vi "SIM_FrameProperties.vi"() -> (0 "data":dbl[][](array[numeric]), 3 "Frame Properties":T1)   [LabVIEW 2019]
uses:
  <vilib>/Utility/file.llb/Read Delimited Spreadsheet (DBL).vi
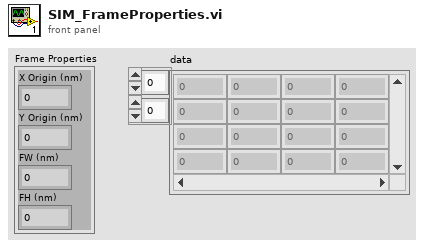
[diagram p1: front panel]
types:
  T1 = cluster{"X Origin (nm)":dbl, "Y Origin (nm)":dbl, "FW (nm)":dbl, "FH (nm)":dbl}
  T2 = cluster{"[0]":dbl, "[1]":dbl, "[2]":dbl, "[3]":dbl, "[4]":dbl, "[5]":dbl, "[6]":dbl, "[7]":dbl, "[8]":dbl}
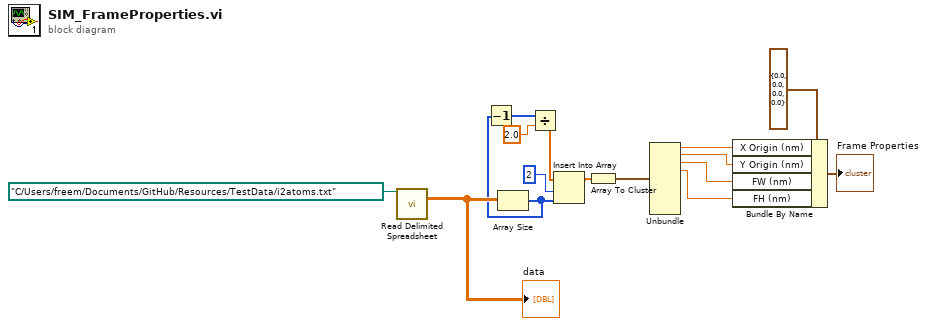
[diagram p0: block diagram]
diagram:
  n1 = call-poly <vilib>:"Read Delimited Spreadsheet.vi"("file path (dialog if empty)"=path "C:/Users/freem/Documents/GitHub/Resources/TestData/i2atoms.txt") -> ("all rows"=w14:dbl[][])  [unwired: 9 in, 5 out]
  "data" <- w14
  n2 = Array Size(array=w14) -> (size(s)=w2:i32[])
  n3 = Decrement(x=w2) -> (x-1=w4:i32[])
  n4 = Divide(x=w4, y=2.0) -> (x/y=w1:dbl[])
  n5 = Insert Into Array(array=w1, index=2, new element=w2) -> (w12:dbl[])
  n6 = Array To Cluster(array=w12) -> (cluster=w11:T2)
  n7 = Unbundle(w11) -> ("[0]"=w9:dbl, "[1]"=w8:dbl, "[2]"=w7:dbl, "[3]"=w6:dbl)  [unwired: 5 out]
  n8 = Bundle By Name(cluster=T1 {"X Origin (nm)"=0.0, "Y Origin (nm)"=0.0, "FW (nm)"=0.0, "FH (nm)"=0.0} ("Frame Properties (Remapped)"), "X Origin (nm)"=w9, "Y Origin (nm)"=w8, "FW (nm)"=w7, "FH (nm)"=w6) -> (→"Frame Properties":T1)
